vi "CommandK.vi"(0 "Keyence":T2={"Serial port sem"=refnum, "Serial port handle"="", "Baud rate"=9600}, 2 "Command":string, 5 "error in":errorcluster) -> (11 "Command time, ms":u32, 14 "Keyence out":T2={"Serial port sem"=refnum, "Serial port handle"="", "Baud rate"=9600}, 16 "Answer":string, 19 "error out":errorcluster)   [LabVIEW 2018]
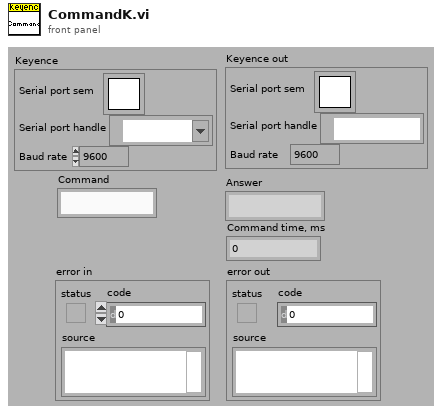
[diagram p1: front panel]
types:
  T1 = typedef "Semaphore RefNum" = refnum<k1>
  T2 = cluster{"Serial port sem":T1, "Serial port handle":refnum<visa-resource-name>, "Baud rate":u32}
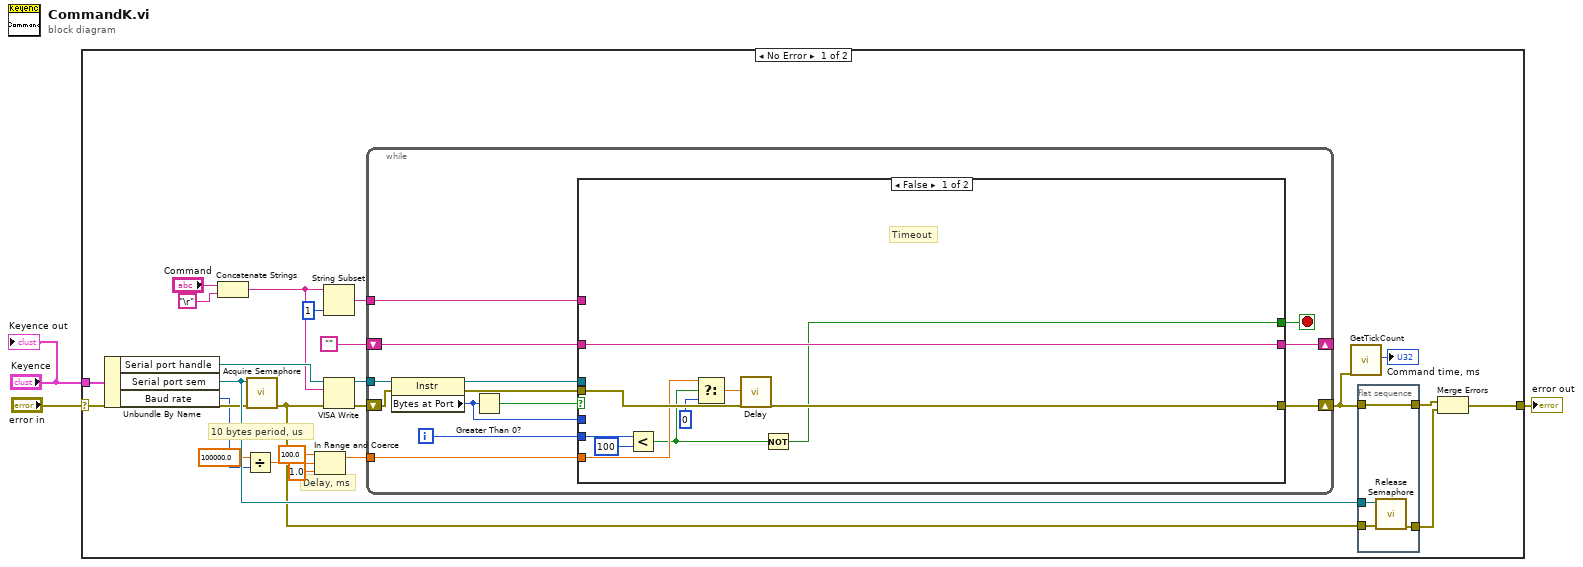
[diagram p0: block diagram]
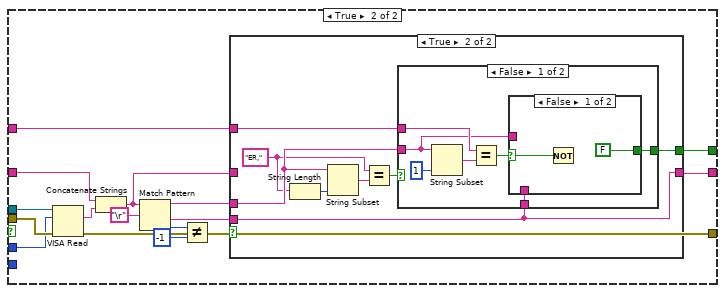
[diagram p2: hidden frame]
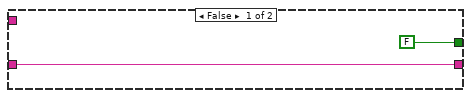
[diagram p3: hidden frame]
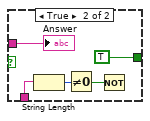
[diagram p4: hidden frame]
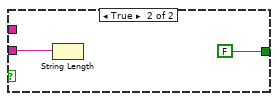
[diagram p5: hidden frame]
diagram:
  n1 = case shown="No Error" "error in" {
    selector: "error in" -> [w23 w97]
    tunnel: [w25 w97] -> w2
    tunnel: "Keyence" -> [w22 _]
    frame No Error {
      # "Delay, ms"
      # "10 bytes period, us"
      n2 = Unbundle By Name(w22) -> ("Serial port handle"=w21:refnum<visa-resource-name>, "Serial port sem"=w24:T1, "Baud rate"=w15:u32)
      n3 = Concatenate Strings("Command", "\r") -> (w7:string)
      n4 = Divide(x=100000.0, y=w15) -> (x/y=w12:dbl)
      n5 = call <vilib>:"Acquire Semaphore.vi"("error in (no error)"=w23, "semaphore"=w24) -> ("error out"=w6:errorcluster)  [unwired: 3 in, 2 out]
      n6 = In Range and Coerce(upper limit=100.0, x=w12, lower limit=1.0) -> (coerced(x)=w11:dbl)  [unwired: 1 out]
      n7 = String Subset(string=w7, length (rest)=1 ("length (rest)")) -> (substring=w17:string)  [unwired: 1 in]
      n8 = VISA Write(VISA resource name=w21, write buffer=w7, error in (no error)=w6) -> (VISA resource name out=w20:refnum<visa-resource-name>, error out=w19:errorcluster)  [unwired: 1 out]
      n9 = while {
        tunnel: w20 -> [w37]
        shift-right: [w34] -> w4
        shift-left: w19 -> [w35]
        tunnel: w17 -> [w32]
        shift-right: [w30] -> _
        shift-left: "" -> [w31]
        tunnel: w11 -> [w29]
        i -> [w28]
        stop <- w36 stop-if-true
        n10 = property class="Instr"(reference=w37, error in=w35) -> (reference out=w39:refnum<visa-resource-name>, error out=w40:errorcluster, "Bytes at Port"=w33:u32)
        n11 = Greater Than 0?(x=w33) -> (x > 0?=w38:bool)
        n12 = case shown="False" w38 {
          tunnel: w39 -> [_ w66]
          tunnel: w40 -> [w50 w65]
          tunnel: w33 -> [_ w64]
          tunnel: [w41 w58] -> w36
          tunnel: [w49 w61] -> w34
          tunnel: w28 -> [w44 _]
          tunnel: w32 -> [_ w60]
          tunnel: w31 -> [w47 w54]
          tunnel: [w47 w51] -> w30
          tunnel: w29 -> [w46 _]
          frame False {
            # "Timeout"
            n13 = Less?(x=w44, y=100 ("x")) -> (x < y?=w42:bool)
            n14 = Select(t=w46, s=w42, f=u32 0 ("Delay")) -> (s? t:f=w48:dbl)
            n15 = call "Delay.vi"("Delay, ms"=w48, "error in"=w50) -> ("error out"=w49:errorcluster)  [unwired: 17 in]
            n16 = Not(x=w42) -> (.not. x?=w41:bool)
          }
          frame True {
            n17 = VISA Read(VISA resource name=w66, byte count=w64, error in (no error)=w65) -> (read buffer=w63:string, error out=w61:errorcluster)  [unwired: 2 out]
            n18 = Concatenate Strings(w54, w63) -> (w53:string)
            n19 = Match Pattern(string=w53, regular expression="\r") -> (before substring=w59:string, after substring=w52:string, offset past match=w57:i32)  [unwired: 1 in, 1 out]
            n20 = Not Equal?(x=w57, y=-1) -> (x != y?=w55:bool)
            n21 = case shown="True" w55 {
              tunnel: w60 -> [_ w74]
              tunnel: w59 -> [_ w73]
              tunnel: w52 -> [_ w69]
              tunnel: [FALSE w72] -> w58
              tunnel: [w68 w69] -> w51
              tunnel: w53 -> [w68 _]
              frame False {
              }
              frame True {
                w71 = "ER," ("string")
                n22 = String Length(string=w71) -> (length=w70:i32)
                n23 = String Subset(string=w73, length (rest)=w70) -> (substring=w76:string)  [unwired: 1 in]
                n24 = Equal?(x=w71, y=w76) -> (x = y?=w75:bool)
                n25 = case shown="False" w75 {
                  tunnel: w74 -> [w81 _]
                  tunnel: w73 -> [w78 w92]
                  tunnel: w69 -> [w79 _]
                  tunnel: [w77 FALSE] -> w72
                  frame False {
                    n26 = String Subset(string=w78, length (rest)=1 ("length (rest)")) -> (substring=w83:string)  [unwired: 1 in]
                    n27 = Equal?(x=w81, y=w83) -> (x = y?=w80:bool)
                    n28 = case shown="False" w80 {
                      selector: w80 -> [w85 _]
                      tunnel: w79 -> [_ w90]
                      tunnel: w78 -> [_ w87]
                      tunnel: [FALSE TRUE] -> w77
                      frame False {
                        n29 = Not(x=w85) -> ()  [unwired: 1 out]
                      }
                      frame True {
                        n30 = String Length(string=w90) -> (length=w89:i32)
                        n31 = Not Equal To 0?(x=w89) -> (x != 0?=w88:bool)
                        n32 = Not(x=w88) -> ()  [unwired: 1 out]
                        "Answer" <- w87
                      }
                    }
                  }
                  frame True {
                    n33 = String Length(string=w92) -> ()  [unwired: 1 out]
                  }
                }
              }
            }
          }
        }
      }
      n34 = call "GetTickCount.vi"("error in (no error)"=w4) -> ("ms"=→"Command time, ms":u32)  [unwired: 17 in, 1 out]
      n35 = flat-sequence {
        tunnel: w6 -> [w96]
        tunnel: w24 -> [w95]
        tunnel: [w94] -> w27
        tunnel: w4 -> [w94]
        tunnel: [w93] -> w26
        frame #0 {
          n36 = call <vilib>:"Release Semaphore.vi"("error in (no error)"=w96, "semaphore"=w95) -> ("error out"=w93:errorcluster)  [unwired: 4 in, 1 out]
        }
      }
      n37 = Merge Errors(w27, w26) -> (w25:errorcluster)
    }
    frame Error {
    }
  }
  "error out" <- w2
  "Keyence out" <- "Keyence"
